vi "RPM to Template.vi"(5 "reset? (True)":bool=TRUE, 8 "window info":T2={"window type"=10, "window length"=2048} {"window type" items=["None"=0, "Hanning"=1, "Hamming"=2, "Blackman-Harris"=3, "Exact Blackman"=4, "Blackman"=5, "Flat Top"=6, "4 Term B-Harris"=7, "7 Term B-Harris"=8, "Low Sidelobe"=9, "Gaussian"=62]; "window length" min=0}, 9 "speed profile":T1 {"speed [RPM]" format="%.2f"; "time [s]" format="%.2f"}, 10 "sampling frequency [Hz]":dbl=1.0 format="%.2f", 11 "signal length":i32 min=0) -> (1 "speed profile out":T1 {"speed [RPM]" format="%.2f"; "time [s]" format="%.2f"}, 3 "Gabor template":dbl[](array[numeric]) format="%.2f")   [LabVIEW 2017, in "SoundVib_Gabor.lvlib"]
doc: "Computes the fundamental frequencies, such as engine rotational speed, in each Gabor window. The fundamental frequency is equal to the first-order instantaneous frequency and is expressed in normalized frequency, f/fs."
uses:
  <vilib>/addons/Sound and Vibration/Order Analysis/Gabor Order Tracking/SoundVib_Gabor.lvlib
  <vilib>/addons/Sound and Vibration/Order Analysis/Tach Process/SubVIs/speed profile.ctl
  <vilib>/addons/Sound and Vibration/Order Analysis/Ref Gabor Order Tracking/window information.ctl
  <vilib>/Analysis/baseanly.llb/Mean (DBL).vi
  <vilib>/Analysis/NI_AALBase.lvlib
  <vilib>/addons/Sound and Vibration/Order Analysis/Tach Process/SoundVib_TachProcess.lvlib
panel:
  # "RPM to Template"
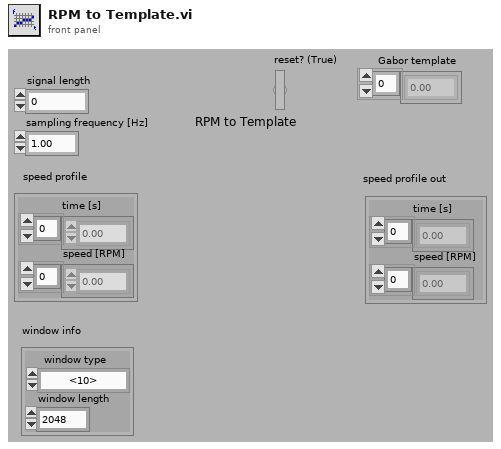
[diagram p1: front panel]
types:
  T1 = typedef "SoundVib_TachProcess.lvlib/speed profile.ctl" = cluster{"time [s]":dbl[], "speed [RPM]":dbl[]}
  T2 = typedef "SoundVib_Gabor.lvlib/window information.ctl" = cluster{"window type":u32, "window length":i32}
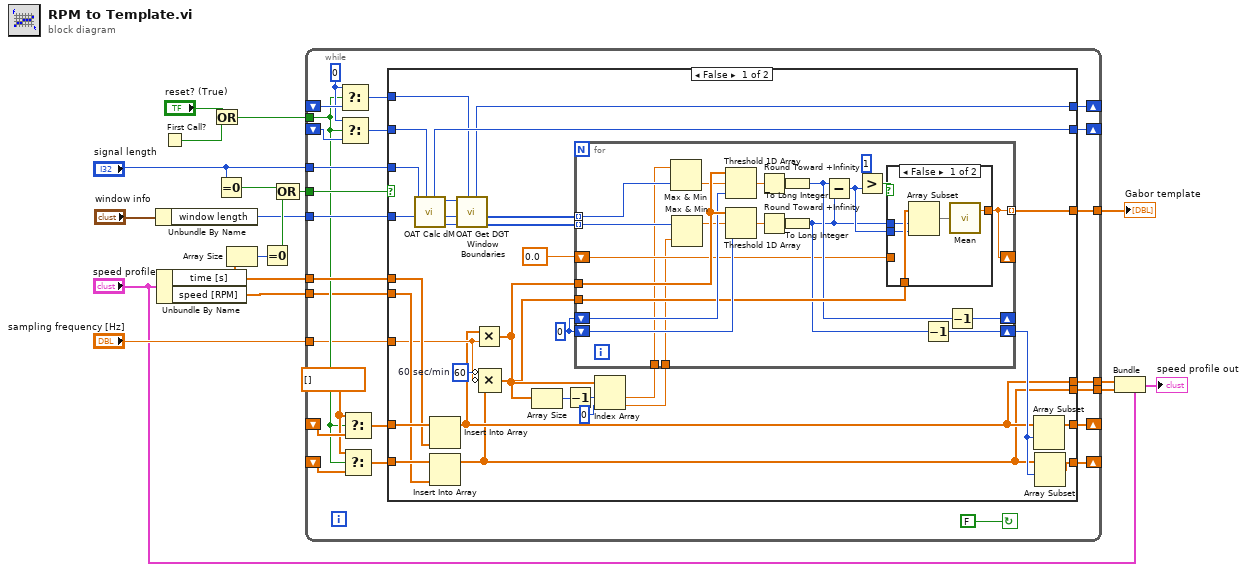
[diagram p0: block diagram]
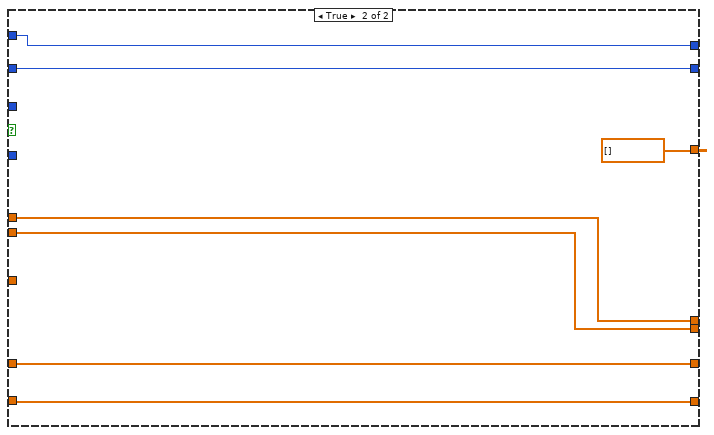
[diagram p3: hidden frame]
diagram:
  n1 = Unbundle By Name("window info") -> ("window length"=w11:i32)
  n2 = Unbundle By Name("speed profile") -> ("time [s]"=w7:dbl[], "speed [RPM]"=w5:dbl[])
  n3 = First Call?() -> (First Call?: T/F=w9:bool)
  n4 = Or(x="reset? (True)", y=w9) -> (x .or. y?=w8:bool)
  n5 = Equal To 0?(x="signal length") -> (x = 0?=w16:bool)
  n6 = Array Size(array=w7) -> (size(s)=w15:i32)
  n7 = Equal To 0?(x=w15) -> (x = 0?=w14:bool)
  n8 = Compound Arithmetic op=OR(w16, w14) -> (w18:bool)
  n9 = while {
    tunnel: [w21] -> w3
    tunnel: [w22] -> w4
    tunnel: w18 -> [w43]
    tunnel: "signal length" -> [w38]
    tunnel: [w42] -> w13
    tunnel: w11 -> [w41]
    shift-right: [w37] -> _
    shift-left: _ -> [w39]
    tunnel: w8 -> [w24]
    shift-right: [w32] -> _
    shift-left: _ -> [w34]
    tunnel: w7 -> [w31]
    tunnel: "sampling frequency [Hz]" -> [w19]
    tunnel: w5 -> [w20]
    shift-right: [w30] -> _
    shift-left: _ -> [w28]
    shift-right: [w29] -> _
    shift-left: _ -> [w25]
    stop <- FALSE continue-if-true
    w26 = dbl[] [] ("t")
    w35 = 0 ("t")
    n10 = Select(t=w35, s=w24, f=w39) -> (s? t:f=w36:i32)
    n11 = Select(t=w35, s=w24, f=w34) -> (s? t:f=w33:i32)
    n12 = Select(t=w26, s=w24, f=w28) -> (s? t:f=w27:dbl[])
    n13 = Select(t=w26, s=w24, f=w25) -> (s? t:f=w23:dbl[])
    n14 = case shown="False" w43 {
      tunnel: w38 -> [w72 _]
      tunnel: w41 -> [w69 _]
      tunnel: w31 -> [w58 w106]
      tunnel: w20 -> [w57 w105]
      tunnel: [w70 dbl[] []] -> w42
      tunnel: w36 -> [w52 w110]
      tunnel: [w51 w110] -> w37
      tunnel: w33 -> [w67 w109]
      tunnel: [w54 w109] -> w32
      tunnel: w23 -> [w60 w107]
      tunnel: w27 -> [w59 w108]
      tunnel: [w50 w108] -> w30
      tunnel: [w56 w107] -> w29
      tunnel: [w47 w106] -> w22
      tunnel: [w44 w105] -> w21
      tunnel: w19 -> [w48 _]
      frame False {
        w49 = 60  # 60 sec/min
        w75 = 0
        n15 = call <vilib>:"OAT Calc dM.vi"("recieved"=w67, "window length"=w69, "signal length"=w72) -> ("dM"=w66:i32, "actual window length"=w64:i32, "# of Gabor windows"=w65:i32, "left"=w54:i32)  [unwired: 5 in]
        n16 = Insert Into Array(array=w59, new element=w58) -> (w47:dbl[])  [unwired: 1 in]
        n17 = Insert Into Array(array=w60, new element=w57) -> (w44:dbl[])  [unwired: 1 in]
        n18 = call <vilib>:"OAT Get DGT Window Boundaries.vi"("offset"=w52, "dM"=w66, "actual window length"=w64, "# of Gabor windows"=w65) -> ("start positions"=w62:i32[], "end positions"=w63:i32[], "next offset"=w51:i32)  [unwired: 5 in]
        n19 = Multiply(x=w47, y=w48) -> (x*y=w46:dbl[])
        n20 = Compound Arithmetic op=MULTIPLY(invert w49, invert w48, w44) -> (w45:dbl[])
        n21 = Array Size(array=w46) -> (size(s)=w74:i32)
        n22 = Decrement(x=w74) -> (x-1=w73:i32)
        n23 = Index Array(array=w46, index #1=w73, index #2=0 ("Index")) -> (element #1=w53:dbl, element #2=w61:dbl)
        n24 = for {
          shift-right: [w83] -> _
          shift-left: w75 -> [w96]
          tunnel: [w80] -> w70 mode=indexing
          tunnel: w46 -> [w98]
          shift-right: [w82] -> w55
          shift-left: w75 -> [w97]
          tunnel: w45 -> [w93]
          shift-right: [w80] -> _
          shift-left: 0.0 -> [w81]
          tunnel: w63 -> [w79] mode=indexing
          tunnel: w62 -> [w78] mode=indexing
          tunnel: w61 -> [w77]
          tunnel: w53 -> [w76]
          n25 = Max & Min(x=w76, y=w79) -> (min(x,y)=w95:dbl)  [unwired: 1 out]
          n26 = Max & Min(x=w78, y=w77) -> (max(x,y)=w94:dbl)  [unwired: 1 out]
          n27 = Threshold 1D Array(1:w96, 2:w95, 3:w98) -> (0:w92:dbl)
          n28 = Threshold 1D Array(1:w97, 2:w94, 3:w98) -> (0:w90:dbl)
          n29 = Round Toward +Infinity(x=w92) -> (ceil(x): smallest int >= x=w87:dbl)
          n30 = Round Toward +Infinity(x=w90) -> (ceil(x): smallest int >= x=w86:dbl)
          n31 = To Long Integer(number=w87) -> (32bit integer=w85:i32)
          n32 = To Long Integer(number=w86) -> (32bit integer=w84:i32)
          n33 = Subtract(x=w85, y=w84) -> (x-y=w91:i32)
          n34 = Greater?(x=1, y=w91) -> (0:w88:bool)
          n35 = case shown="False" w88 {
            tunnel: w93 -> [w103 _]
            tunnel: w91 -> [w102 _]
            tunnel: [w101 w104] -> w80
            tunnel: w84 -> [w99 _]
            tunnel: w81 -> [_ w104]
            frame False {
              n36 = Array Subset(array=w103, index=w99, length=w102) -> (w100:dbl[])
              n37 = call-poly <vilib>:"Mean.vi"("X"=w100) -> ("mean"=w101:dbl)  [unwired: 1 out]
            }
            frame True {
            }
          }
          n38 = Decrement(x=w84) -> (x-1=w82:i32)
          n39 = Decrement(x=w85) -> (x-1=w83:i32)
        }
        n40 = Array Subset(array=w47, index=w55) -> (w50:dbl[])  [unwired: 1 in]
        n41 = Array Subset(array=w44, index=w55) -> (w56:dbl[])  [unwired: 1 in]
      }
      frame True {
      }
    }
  }
  "Gabor template" <- w13
  n42 = Bundle(cluster="speed profile", "time [s]"=w4, "speed [RPM]"=w3) -> (→"speed profile out":T1)
